vi "Register Groups.vi"(8 "error in (no error)":errorcluster, 9 "Promise":refnum<class "Promise.lvclass">, 10 "Groups":refnum<class "Group.lvclass">[](array[class]), 11 "DataHandler in":refnum<class "DataHandler.lvclass">) -> (0 "error out":errorcluster, 3 "DataHandler out":refnum<class "DataHandler.lvclass">)   [LabVIEW 2020, in "VolatusData.lvlib" / "DataHandler.lvclass"]
uses:
  DataHandler.lvclass
  lv-vecto/Vecto/Group/Group.lvclass
  lv-promises/Promises/Promise/Promise.lvclass
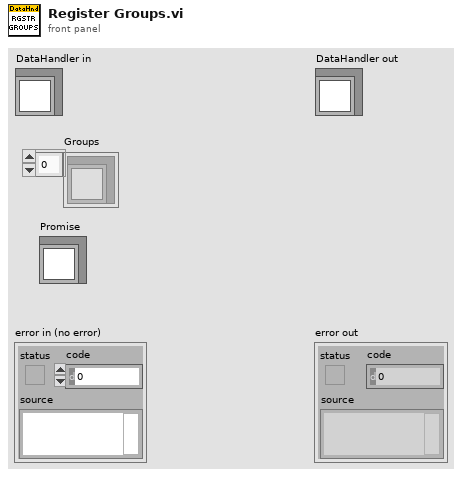
[diagram p1: front panel]
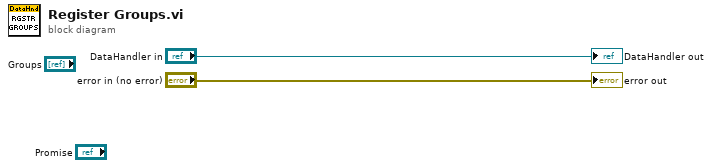
[diagram p0: block diagram]
diagram:
  "error out" <- "error in (no error)"
  "DataHandler out" <- "DataHandler in"
